vi "Insert SubPanel.vi"(8 "error in (no error)":errorcluster, 10 "VI Ref":refnum<vi>, 11 "Subpanel Ref":refnum<vi>) -> (0 "error out":errorcluster)   [LabVIEW 2015]
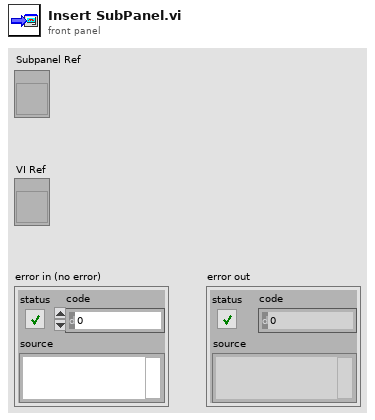
[diagram p1: front panel]
types:
  T1 = enum32{"Invalid", "Standard", "Closed", "Hidden", "Minimized", "Maximized"}
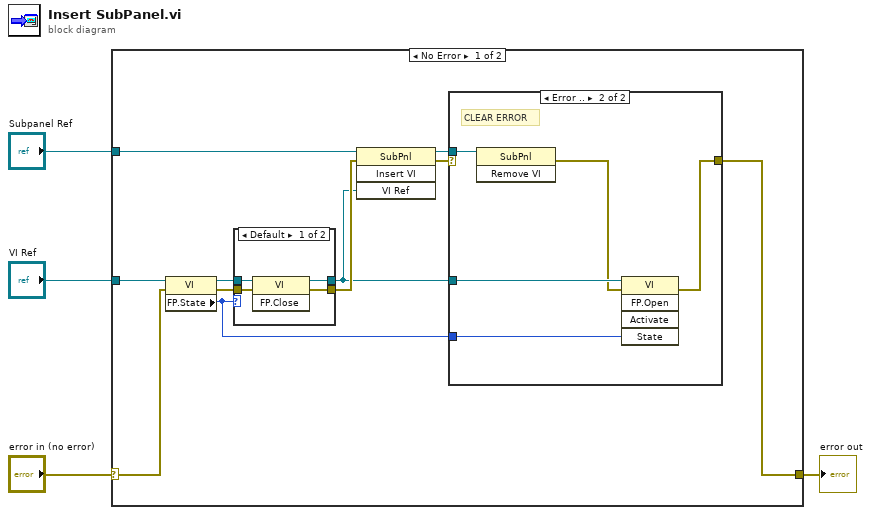
[diagram p0: block diagram]
diagram:
  n1 = case shown="No Error" "error in (no error)" {
    selector: "error in (no error)" -> [w6 w28]
    tunnel: "VI Ref" -> [w15 _]
    tunnel: "Subpanel Ref" -> [w12 _]
    tunnel: [w5 w28] -> w1
    frame No Error {
      n2 = property class="VI"(reference=w15, error in=w6) -> (reference out=w14:refnum<vi>, error out=w13:errorcluster, "FP.State"=w7:T1)
      n3 = case shown="Default" w7 {
        tunnel: w14 -> [w19 w21]
        tunnel: w13 -> [w18 w20]
        tunnel: [w17 w21] -> w8
        tunnel: [w16 w20] -> w11
        frame Default {
          n4 = invoke class="VI" method="FP.Close"(reference=w19, error in=w18) -> (reference out=w17:refnum<vi>, error out=w16:errorcluster)  [unwired: 1 in, 1 out]
        }
        frame "Closed" {
        }
      }
      n5 = invoke class="SubPnl" method="Insert VI"(reference=w12, error in=w11, "VI Ref"=w8) -> (reference out=w9:refnum<vi>, error out=w10:errorcluster)  [unwired: 1 in, 2 out]
      n6 = case shown="Error .." w10 {
        selector: w10 -> [w22 _]
        tunnel: w9 -> [_ w27]
        tunnel: w8 -> [_ w26]
        tunnel: w7 -> [_ w24]
        tunnel: [w22 w23] -> w5
        frame No Error {
        }
        frame Error {
          # "CLEAR ERROR"
          n7 = invoke class="SubPnl" method="Remove VI"(reference=w27) -> (error out=w25:errorcluster)  [unwired: 2 in, 2 out]
          n8 = invoke class="VI" method="FP.Open"(reference=w26, error in=w25, "State"=w24) -> (error out=w23:errorcluster)  [unwired: 2 in, 4 out]
        }
      }
    }
    frame Error {
    }
  }
  "error out" <- w1
